vi "CENTER.vi"(11 "Cam 0":T1) -> (3 "Numeric":dbl)   [LabVIEW 2020]
uses:
  CamSettingSUB_TypDEf.ctl
  CamAndObj_TypDEf.ctl
  OnOffTypeDef.ctl
  userROI.ctl
  source/Device Drivers/shared/numericVariable_TypeDef.ctl
  CamRoiTypDef.ctl
  source/Device Drivers/BaseDriver/BaseDriver.lvclass
panel:
  in  "manual":bool
  in  "manual":dbl
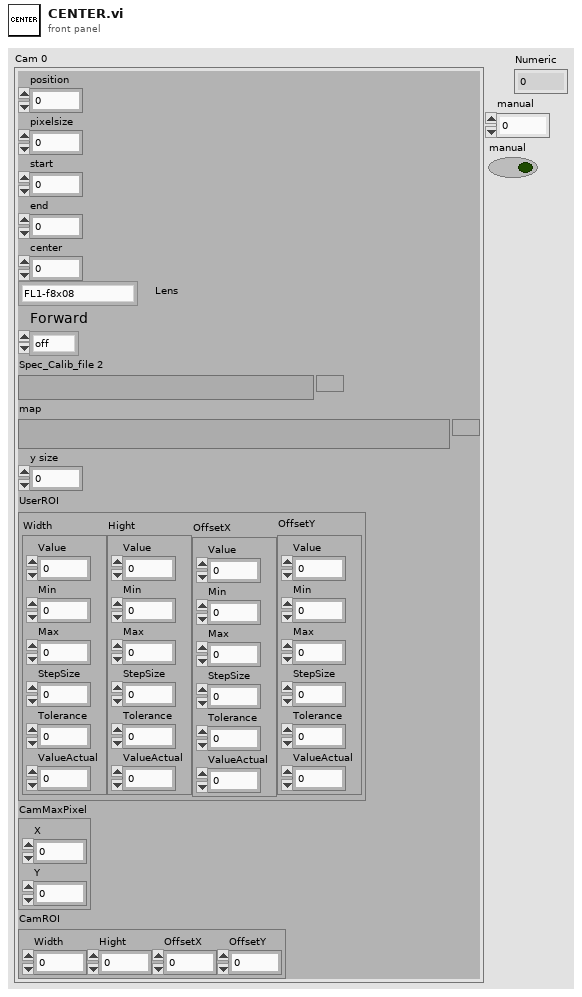
[diagram p1: front panel]
types:
  T1 = typedef "CamSettingSUB_TypDEf.ctl" = cluster{"position":dbl, "pixelsize":dbl, "start":dbl, "end":dbl, "center":dbl, "Lens":T2, "Forward":T3, "Spec_Calib_file 2":path, "map":path, "y size":i32, "UserROI":T4, "CamMaxPixel":cluster{"X":i32, "Y":i32}, "CamROI":T6}
  T2 = typedef "CamAndObj_TypDEf.ctl" = enum16{"FL1-f8x08", "FL1-f8x06", "FL1-f8", "ch300-f50", "FL2G-f8", "FL3M14-f8", "FL3M14-f8x08", "FL3M14-f8x08(2x2)"}
  T3 = typedef "OnOffTypeDef.ctl" = enum16{"off", "on"}
  T4 = typedef "userROI.ctl" = cluster{"Width":T5, "Hight":T5, "OffsetX":T5, "OffsetY":T5}
  T5 = typedef "BaseDriver.lvclass/numericVariable_TypeDef.ctl" = cluster{"Value":dbl, "Min":dbl, "Max":dbl, "StepSize":dbl, "Tolerance":dbl, "ValueActual":dbl}
  T6 = typedef "CamRoiTypDef.ctl" = cluster{"Width":dbl, "Hight":dbl, "OffsetX":dbl, "OffsetY":dbl}
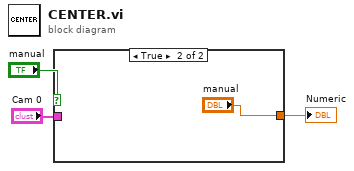
[diagram p0: block diagram]
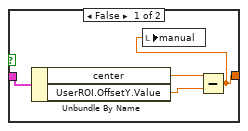
[diagram p2: hidden frame]
diagram:
  n1 = case shown="True" "manual" {
    tunnel: [w4 "manual"] -> w3
    tunnel: "Cam 0" -> [w5 _]
    frame False {
      n2 = Unbundle By Name(w5) -> ("center"=w6:dbl, "UserROI.OffsetY.Value"=w7:dbl)
      n3 = Subtract(x=w6, y=w7) -> (x-y=w4:dbl)
      n4 = local write "manual"(w4) -> ()
    }
    frame True {
    }
  }
  "Numeric" <- w3
